vi "Calibration.vi"(0 "Mode":T3, 5 "Calib file":path, 9 "Simulate/Run":T2) -> (14 "Calib const":string[][](array[string]), 16 "Coefficients":dbl[][](array[numeric]) format="%.2f", 19 "Status Out":T1)   [LabVIEW 2013]
uses:
  Anemometry Sub Vis/Globals/Calib_global.vi
  Anemometry Sub Vis/Globals/Meas_global.vi
  Anemometry Sub Vis/Controls/Setup.ctl
  Anemometry Sub Vis/Controls/Post_Process.ctl
  Anemometry Sub Vis/Gen Trav/Multi_Run_Status.ctl
  Anemometry Sub Vis/Controls/App_Global.ctl
  Anemometry Sub Vis/Calibration/Calib_mode.ctl
  Anemometry Sub Vis/Controls/Save_Data.ctl
  Anemometry Sub Vis/Acquisition/PWA/PWAtasksGLOBAL.vi
  Anemometry Sub Vis/File/Setup_Filetype.ctl
  <vilib>/Analysis/NI_AALBase.lvlib
  <vilib>/Analysis/baseanly.llb/Mean (DBL).vi
  Anemometry Sub Vis/Controls/User_Specific_mode.ctl
panel:
  in  "-ve Ref Values":bool
  out "String":string
  in  "polynomial order":i32=2 min=1 max=3 step=1
  out "Ref velocity":dbl[](array[numeric])=[2.4275346736, 2.4395664609, 2.453235235, 2.4247395837, 2.4277603784, 2.41169823, 2.4254144559, 2.424896502176921] format="%.3f"
  out "labels":string[](array[string])=["XW1 Volt", "XW2 Volt", "Entered Val", "Selector"]
  in  "Point selector 3":cluster{"Y":dbl, "X":dbl, "t/f":bool}[](array[cluster]) {"X" format="%#.2g"; "Y" format="%#.3f"}
  in  "n":dbl=0.45 format="%.4f"
  in  "Fixed n":bool=TRUE
  out "Sample of input signals":dbl[][](graph)
  in  "Sampling speeds":T4={"Samples/ch"=600, "Sample Rate/ch (Hz)"=100.0} {"Sample Rate/ch (Hz)" min=0; "Samples/ch" min=0 step=1}
  out "Calibration plot":cluster{cluster{dbl, dbl}[]}[](graph)
  in  "Point selector 4":T5(array[cluster]) {"Y2" format="%#.2f"; "X" format="%#.3f"; "Y" format="%#.2f"}
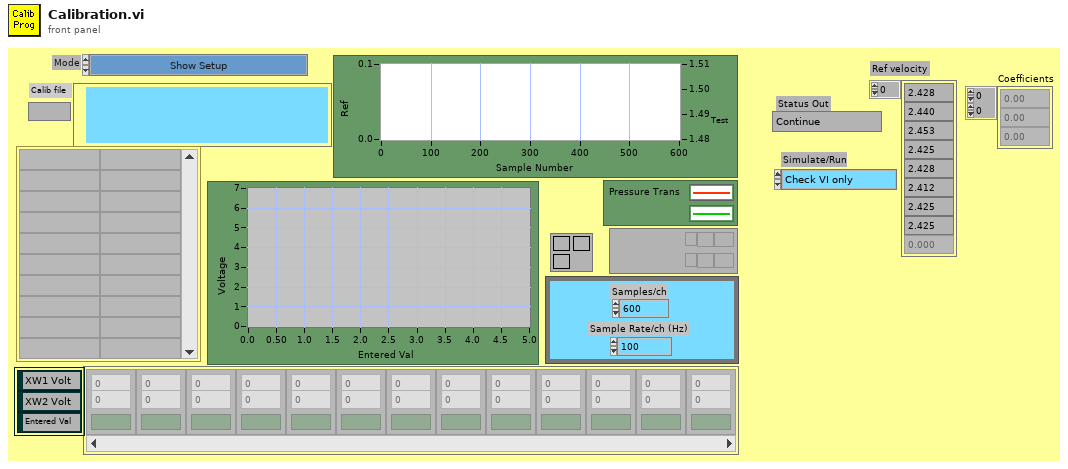
[diagram p1: front panel]
types:
  T1 = typedef "Multi_Run_Status.ctl" = enum16{"Continue", "Jump to Next Point", "Jump to Next Row", "Jump To Fall Back", "Terminate Run"}
  T2 = typedef "User_Specific_mode.ctl" = enum16{"Check VI only", "Run VI"}
  T3 = typedef "Calib_mode.ctl" = enum16{"Show Setup", "Take a New Calibration Point", "Refit Curve", "Setup Front Panel"}
  T4 = cluster{"Samples/ch":i32, "Sample Rate/ch (Hz)":sgl}
  T5 = cluster{"Y":dbl, "Y2":dbl, "X":dbl, "t/f":bool}[]
  T6 = typedef "Post_Process.ctl" = enum16{"Take New Data", "Post Process Raw Data File"}
  T7 = typedef "Setup_Filetype.ctl" = enum16{"Measurement Setups", "Calibration Setups", "General", "Results File Plotter Setups", "Speed Calib Tweaks"}
  T8 = typedef "Save_Data.ctl" = enum16{"Save No Data", "Save Data"}
  T9 = typedef "Setup.ctl" = enum16{"Run Program", "Show Setup", "Save Current Setup", "Setup Front Panel"}
  T10 = typedef "App_Global.ctl" = enum16{"Read Global", "Write to Global", "Initialise Array"}
  T11 = enum32{"existing file", "new file", "new or existing file", "existing dir", "new dir", "new or existing dir", "existing file (use LLBs)", "new file (use LLBs)", "new or existing file (use LLBs)", "new or existing file or directory (use LLBs)"}
  T12 = cluster{"Samples /ch":i32, "Sampling Rate /ch (Hz)":sgl}
  T13 = typedef "Cal_Inst_type.ctl" = enum16{"Propeller anemometer", "Pressure Transducer", "Hot wire", "Cross wire velocity", "Cross wire angle", "Generic Linear", "Generic Polynomial", "Generic BackPoly", "Fast FID", "Thermocouple", "Cold wire", "Pulsed Wire"}
  T14 = typedef "Ref_Inst_type.ctl" = enum16{"Propellor anemometer", "Pressure Transducer", "Raw voltage", "Pitot-static tube", "Preston tube", "Generic Linear", "Generic Polynomial", "Thermocouple", "LDA", "Enter Value", "ADAM Channel"}
  T15 = cluster{"2nd Ref type":T14, "2nd inst present":bool}
  T16 = typedef "Analysis_info_cluster.ctl" = cluster{"Colour":u32, "Inst type":T17, "Inst name":string, "Symbol":string, "Code name":string, "Extra Info":string, "Inst Array":T18, "Extra Titles":string[], "Extra Values":string[], "U":dbl, "u^2":dbl, "u^3":dbl, "u^4":dbl, "Skew_u":dbl, "Kurt_u":dbl, "Sd Error in Mean":dbl, "% u'/U":dbl, "X":dbl, "Y":dbl, "Z":dbl, "Timescale integral to 25%":dbl, "Sd Error in Variance":dbl, "Calib File":path, "Calib Constants":dbl[], "Output Position":bool, "Full Stats":bool, "Av Sampling Rate":dbl, "Av No of Samples":dbl, "Total Meas Time (s)":dbl, "ADAM Ch Name":string}
  T17 = typedef "Inst_type.ctl" = enum16{"Propeller anemometer", "Raw voltage", "Pressure Transducer", "Pitot-static tube", "Preston tube", "Hot wire", "Cross wire 1", "Cross wire 2", "Generic Linear", "Generic Polynomial", "Generic BackPoly", "Fast FID", "Thermocouple", "Cold wire", "Pulsed Wire", "LDA Vel", "LDA Tran time", "LDA Arr time"}
  T18 = typedef "Instrument_Array.ctl" = enum16{"PWA", "LDA", "Analogue"}
  T19 = typedef "Time_Trace_Cluster.ctl" = cluster{"Weighting":dbl[], "Time (s)":dbl[], "Voltage":dbl[], "Eng Values":dbl[]}
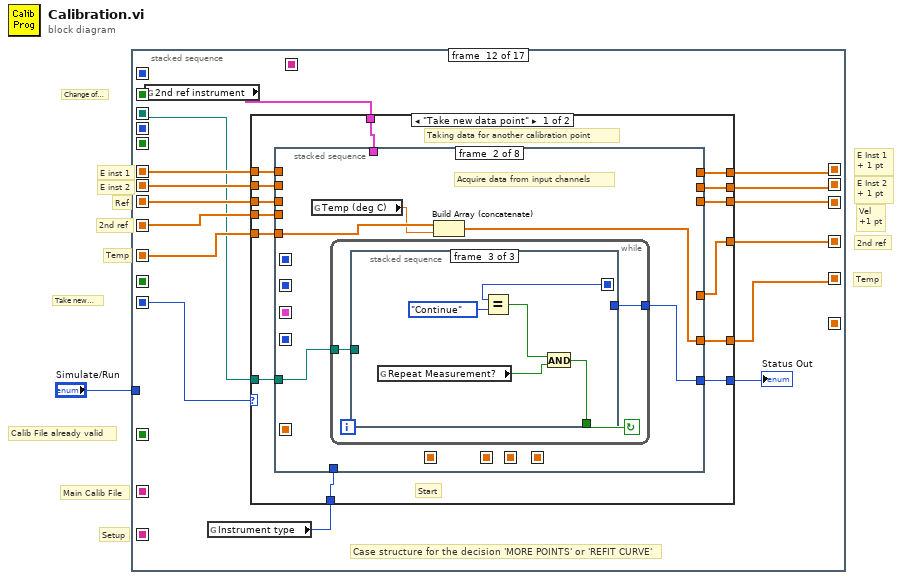
[diagram p0: block diagram]
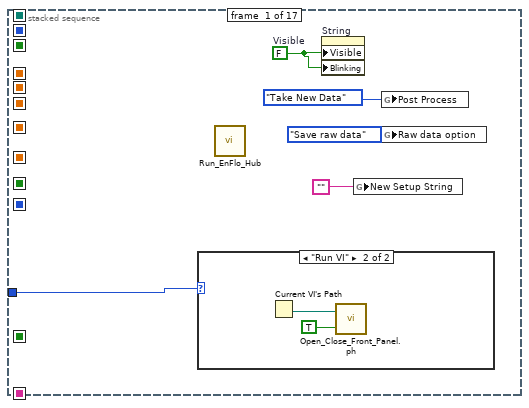
[diagram p2: hidden frame]
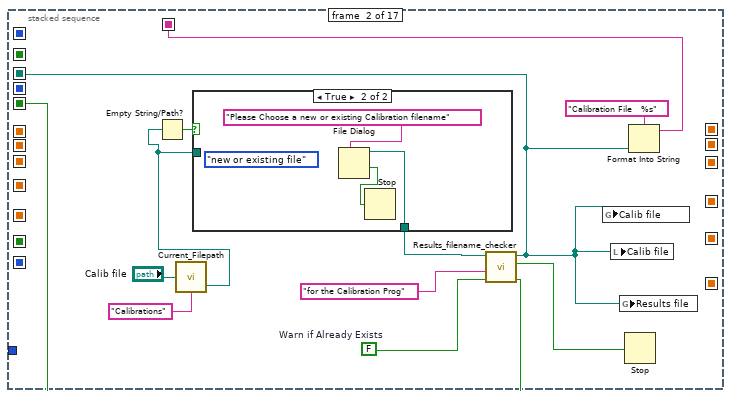
[diagram p4: hidden frame]
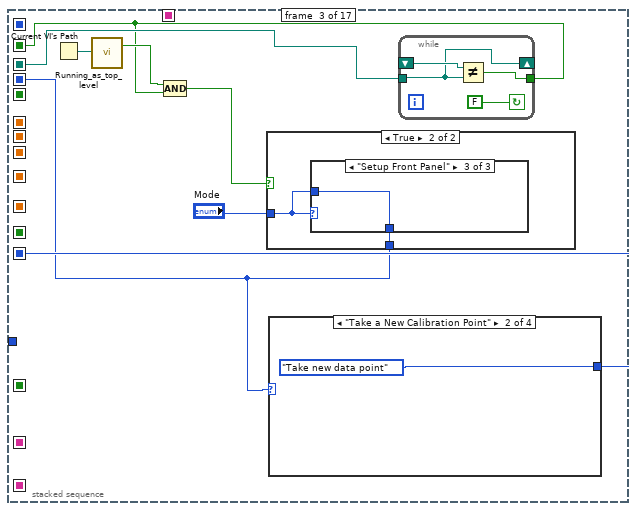
[diagram p6: hidden frame]
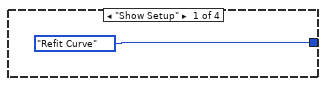
[diagram p7: hidden frame]
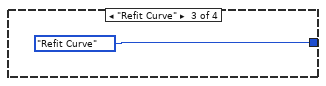
[diagram p8: hidden frame]
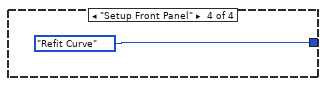
[diagram p9: hidden frame]
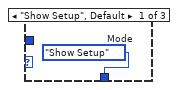
[diagram p11: hidden frame]
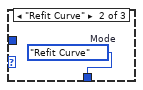
[diagram p12: hidden frame]
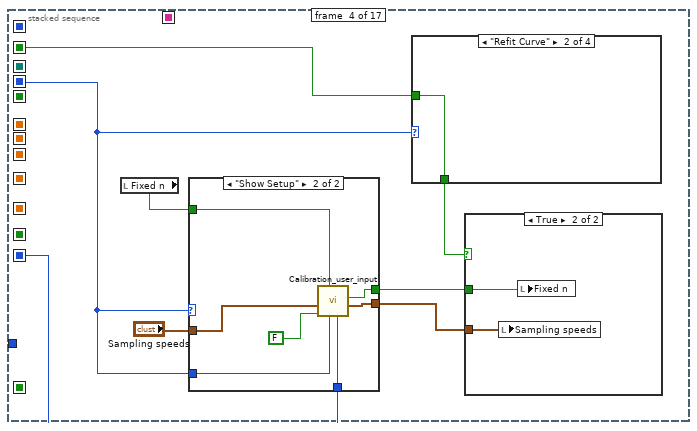
[diagram p13: hidden frame]
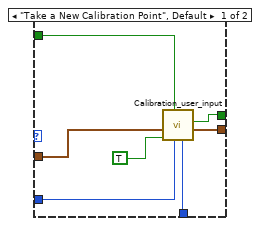
[diagram p14: hidden frame]
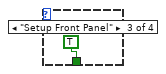
[diagram p16: hidden frame]
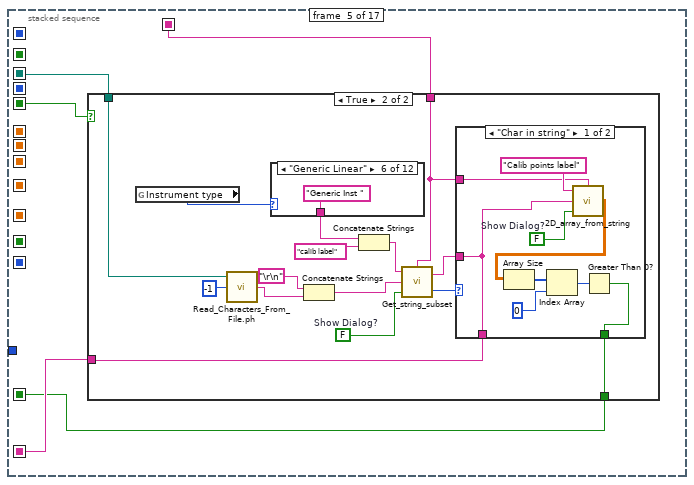
[diagram p19: hidden frame]
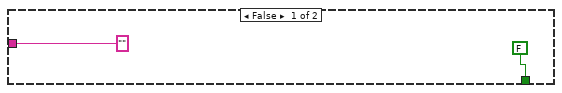
[diagram p20: hidden frame]
diagram:
  # "Change of file"
  # "Take new point"
  # "Calib File already valid"
  # "Main Calib File"
  # "Temp"
  # "Temp"
  # "Setup"
  # "E inst 1"
  # "Ref"
  # "E Inst 1\n+ 1 pt"
  # "Vel\n+1 pt"
  # "E inst 2"
  # "E Inst 2\n+ 1 pt"
  # "2nd ref"
  # "2nd ref"
  n1 = stacked-sequence {
    seq-local: [_ _ _ _ _ _ _ _ _ _ _ w489 _ _ _ _ _] -> [_ _ _ _ _ _ _ _ _ _ _ _ w683 _ _ _ _]
    seq-local: [_ _ _ _ _ _ _ _ _ _ _ w488 _ _ _ _ _] -> [_ _ _ _ _ _ _ _ _ _ _ _ w686 _ _ w749 _]
    seq-local: [_ _ _ _ _ _ _ w376 _ _ _ _ _ _ _ _ _] -> [_ _ _ _ _ _ _ _ _ _ _ w491 _ _ _ _ _]
    seq-local: [_ _ _ _ _ _ _ w375 _ _ _ _ _ _ _ _ _] -> [_ _ _ _ _ _ _ _ _ _ _ w490 _ _ _ _ _]
    seq-local: [_ _ _ _ _ _ _ w374 _ _ _ _ _ _ _ _ _] -> [_ _ _ _ _ _ _ _ _ _ _ w486 _ _ _ _ _]
    seq-local: [_ _ _ _ _ _ _ _ _ _ _ w487 _ _ _ _ _] -> [_ _ _ _ _ _ _ _ _ _ _ _ w685 _ _ _ _]
    seq-local: [_ _ _ _ _ _ _ w373 _ _ _ _ _ _ _ _ _] -> [_ _ _ _ _ _ _ _ _ _ _ w485 _ _ _ _ _]
    seq-local: [_ _ _ _ _ _ _ _ _ _ _ w484 _ _ _ _ _] -> [_ _ _ _ _ _ _ _ _ _ _ _ w680 _ _ _ _]
    seq-local: [_ _ _ _ w78 _ _ _ _ _ _ _ _ _ _ _ _] -> [_ _ _ _ _ _ _ w362 _ _ _ _ _ _ _ _ _]
    seq-local: [_ _ _ _ w79 _ _ _ _ _ _ _ _ _ _ _ _] -> [_ _ _ _ _ _ _ w363 _ _ _ _ _ _ _ _ _]
    seq-local: [_ _ _ _ _ _ _ _ _ _ w464 _ _ _ _ _ _] -> [_ _ _ _ _ _ _ _ _ _ _ _ _ _ w727 _ _]
    seq-local: [_ _ _ _ _ _ _ _ _ _ _ w482 _ _ _ _ _] -> [_ _ _ _ _ _ _ _ _ _ _ _ w684 _ _ _ _]
    seq-local: [_ _ _ _ _ _ _ w372 _ _ _ _ _ _ _ _ _] -> [_ _ _ _ _ _ _ _ _ _ _ w481 _ _ _ _ _]
    seq-local: [_ w13 _ _ _ _ _ _ _ _ _ _ _ _ _ _ _] -> [_ _ w29 _ w77 _ _ _ _ _ w465 w479 _ w709 w736 w750 _]
    seq-local: [_ w18 _ _ _ _ _ _ _ _ _ _ _ _ _ _ _] -> [_ _ _ _ w76 _ _ _ w405 _ _ _ _ _ _ _ _]
    seq-local: [_ _ w32 _ _ _ _ _ _ _ _ _ _ _ _ _ _] -> [_ _ _ w50 _ _ _ _ _ _ _ w478 _ _ _ w751 _]
    seq-local: [_ _ w25 _ _ _ _ _ _ _ _ _ _ _ _ _ _] -> [_ _ _ w49 _ _ _ _ _ w422 _ _ _ _ _ _ w793]
    seq-local: [_ _ _ _ _ _ _ w364 _ _ _ _ _ _ _ _ _] -> [_ _ _ _ _ _ _ _ w403 _ _ _ _ _ _ _ _]
    seq-local: [_ _ _ _ _ _ _ _ _ _ _ _ w681 _ _ _ _] -> [_ _ _ _ _ _ _ _ _ _ _ _ _ w693 _ _ _]
    seq-local: [_ _ _ _ _ _ _ _ _ _ _ _ w679 _ _ _ _] -> [_ _ _ _ _ _ _ _ _ _ _ _ _ w708 _ _ _]
    seq-local: [_ _ w28 _ _ _ _ _ _ _ _ _ _ _ _ _ _] -> [_ _ _ w47 _ _ _ _ w402 _ _ _ _ _ _ _ _]
    seq-local: [_ w12 _ _ _ _ _ _ _ _ _ _ _ _ _ _ _] -> [_ _ _ _ w75 _ _ w357 _ _ _ _ _ _ _ _ _]
    tunnel: "Simulate/Run" -> [w5 _ _ _ _ _ _ _ _ _ _ _ _ _ _ _ _]
    frame #0 {
      w3 = FALSE  # Visible
      n2 = case shown="\"Run VI\"" w5 {
        frame "Check VI only" {
        }
        frame "Run VI" {
          n3 = Current VI's Path() -> (path=w7:path)
          n4 = call "Open_Close_Front_Panel.ph.vi"("Front Panel Window:Open"=TRUE, "VI path"=w7) -> ()  [unwired: 2 out]
        }
      }
      n5 = call "Run_EnFlo_Hub.vi"() -> ()  [unwired: 8 out]
      n6 = property on="String" class="Str"("Visible"=w3, "Blinking"=w3) -> ()  [unwired: 2 in, 2 out]
      n7 = global write "Calib_global.vi" "New Setup String"("") -> ()
      n8 = global write "Meas_global.vi" "Post Process"(Post_Process."Take New Data" ("Post Process")) -> ()
      n9 = global write "Meas_global.vi" "Raw data option"(enum16{"Save raw data", "Raw data not saved"}."Save raw data" ("Raw data option")) -> ()
    }
    frame #1 {
      w19 = FALSE  # Warn if Already Exists
      n10 = call "Current_Filepath.vi"("Filename in"="Calib file", "Data Type"="Calibrations") -> ("Filename Out"=w10:path)  [unwired: 1 out]
      n11 = Empty String/Path?(string/path=w10) -> (empty?=w15:bool)
      n12 = case shown="True" w15 {
        tunnel: w10 -> [w21 _]
        tunnel: [w21 w23] -> w17
        frame False {
        }
        frame True {
          (unwired) T11."new or existing file" ("select mode (2)")
          n13 = File Dialog(7:"Please Choose a new or existing Calibration filename" ("Promp if not found")) -> (1:w22:bool, 3:w23:path)  [unwired: 1 in, 7 out]
          n14 = Stop(stop? (T)=w22) -> ()
        }
      }
      n15 = call "Results_filename_checker.vi"("Warn if Already Exists"=w19, "Comment"="for the Calibration Prog", "Results file"=w17) -> ("exists?"=w18:bool, "cancelled"=w16:bool, "Results file output"=w13:path)  [unwired: 2 in, 1 out]
      n16 = global write "Calib_global.vi" "Calib file"(w13) -> ()
      n17 = local write "Calib file"(w13) -> ()
      n18 = global write "Meas_global.vi" "Results file"(w13) -> ()
      n19 = Stop(stop? (T)=w16) -> ()
      n20 = Format Into String(format string="Calibration File   %s", w13) -> (resulting string=w12:string)  [unwired: 2 in, 1 out]
    }
    frame #2 {
      n21 = Current VI's Path() -> (path=w31:path)
      n22 = call "Running_as_top_level.vi"("Vi path name"=w31) -> ("Top Level"=w30:bool)  [unwired: 1 out]
      n23 = while {
        shift-right: [w45] -> _
        shift-left: _ -> [w46]
        tunnel: w29 -> [w45]
        tunnel: [w44] -> w28
        stop <- FALSE continue-if-true
        n24 = Not Equal?(x=w46, y=w45) -> (x != y?=w44:bool)
      }
      n25 = Compound Arithmetic op=AND(w30, w28) -> (w27:bool)
      n26 = case shown="True" w27 {
        tunnel: "Mode" -> [w37 w38]
        tunnel: [w37 w39] -> w25
        frame False {
        }
        frame True {
          n27 = case shown="\"Setup Front Panel\"" w38 {
            tunnel: [w40 w41 w42] -> w39
            tunnel: w38 -> [_ _ w42]
            frame "Show Setup", Default {
              w40 = Calib_mode."Show Setup"  # Mode
            }
            frame "Refit Curve" {
              w41 = Calib_mode."Refit Curve"  # Mode
            }
            frame "Setup Front Panel" {
            }
          }
        }
      }
      n28 = case shown="\"Take a New Calibration Point\"" w25 {
        tunnel: [enum16{"Take new data point", "Refit Curve"}."Refit Curve" ("data mode") enum16{"Take new data point", "Refit Curve"}."Take new data point" ("data mode") enum16{"Take new data point", "Refit Curve"}."Refit Curve" ("data mode") enum16{"Take new data point", "Refit Curve"}."Refit Curve" ("data mode")] -> w32
        frame "Show Setup" {
        }
        frame "Take a New Calibration Point" {
        }
        frame "Refit Curve" {
        }
        frame "Setup Front Panel" {
        }
      }
    }
    frame #3 {
      n29 = local read "Fixed n"() -> (w52:bool)
      n30 = case shown="\"Show Setup\"" w49 {
        tunnel: "Sampling speeds" -> [w61 w68]
        tunnel: w49 -> [w59 w66]
        tunnel: w50 -> [w58 w65]
        tunnel: [w57 w64] -> w53
        tunnel: w52 -> [w55 w63]
        tunnel: [w56 w62] -> w51
        frame "Take a New Calibration Point", Default {
          n31 = call "Calibration_user_input.vi"("data mode"=w58, "Mode"=w59, "Fixed n"=w55, "OK"=TRUE, "Sampling speeds"=w61) -> ("Sampling speeds Output"=w57:T12, "Fixed n out"=w56:bool)  [unwired: 2 in, 3 out]
        }
        frame "Show Setup" {
          n32 = call "Calibration_user_input.vi"("data mode"=w65, "Mode"=w66, "Fixed n"=w63, "OK"=FALSE, "Sampling speeds"=w68) -> ("Sampling speeds Output"=w64:T12, "Fixed n out"=w62:bool)  [unwired: 5 out]
        }
      }
      n33 = case shown="\"Refit Curve\"" w49 {
        tunnel: [w69 w70 TRUE w72] -> w48
        tunnel: w47 -> [w69 w70 _ w72]
        frame "Show Setup" {
        }
        frame "Refit Curve" {
        }
        frame "Setup Front Panel" {
        }
        frame "Take a New Calibration Point" {
        }
      }
      n34 = case shown="True" w48 {
        tunnel: w53 -> [_ w74]
        tunnel: w51 -> [_ w73]
        frame False {
        }
        frame True {
          n35 = local write "Sampling speeds"(w74) -> ()
          n36 = local write "Fixed n"(w73) -> ()
        }
      }
    }
    frame #4 {
      n37 = case shown="True" w76 {
        tunnel: ["" ("Output string") w96] -> w79
        tunnel: [FALSE w95] -> w78
        tunnel: w77 -> [_ w87]
        tunnel: w75 -> [_ w82]
        frame False {
        }
        frame True {
          w86 = FALSE  # Show Dialog?
          n38 = global read "Calib_global.vi" "Instrument type"() -> (w90:T13)
          n39 = call "Read_Characters_From_File.ph.vi"("file path (dialog if empty)"=w87, "number of characters (all:-1)"=-1) -> ("character string"=w84:string)  [unwired: 7 out]
          n40 = case shown="\"Generic Linear\"" w90 {
            tunnel: ["Prop " "Mano " "HW " "Cross wire velocity " "Cross wire angle " "Generic Inst " "Generic Polynomial " "Generic BackPoly " "Fast FID " "Thermocouple " "Cold wire " "Pulsed wire "] -> w91
            frame "Propeller anemometer" {
            }
            frame "Pressure Transducer" {
            }
            frame "Hot wire" {
            }
            frame "Cross wire velocity" {
            }
            frame "Cross wire angle" {
            }
            frame "Generic Linear" {
            }
            frame "Generic Polynomial" {
            }
            frame "Generic BackPoly" {
            }
            frame "Fast FID" {
            }
            frame "Thermocouple" {
            }
            frame "Cold wire" {
            }
            frame "Pulsed Wire" {
            }
          }
          n41 = Concatenate Strings("\r\n", w84) -> (w83:string)
          n42 = Concatenate Strings(w91, "calib label") -> (w92:string)
          n43 = call "Get_string_subset.vi"("String Name"=w82, "Show Dialog?"=w86, "String to split"=w83, "File Label"=w92) -> ("Status"=w89:enum16{"Char in string", "Char not in string"}, "Output string"=w88:string)
          n44 = case shown="\"Char in string\"" w89 {
            tunnel: w88 -> [w115 _]
            tunnel: [w115 ""] -> w96
            tunnel: [w110 FALSE] -> w95
            tunnel: w82 -> [w109 _]
            frame "Char in string" {
              w116 = FALSE  # Show Dialog?
              n45 = call "2D_array_from_string.vi"("String Name"=w109, "Show Dialog?"=w116, "Input string"=w115, "Array title"="Calib points label") -> ("2D data array"=w114:dbl[][])
              n46 = Array Size(array=w114) -> (size(s)=w113:i32[])
              n47 = Index Array(array=w113, index=0 ("Index")) -> (element=w111:i32)
              n48 = Greater Than 0?(x=w111) -> (x > 0?=w110:bool)
            }
            frame "Char not in string" {
            }
          }
        }
      }
    }
    frame #5 {
      w122 = ""
      n49 = global read "Calib_global.vi" "2nd ref instrument"() -> (w129:T15)
      n50 = global read "Calib_global.vi" "Ref Instrument type"() -> (w130:T14)
      n51 = Unbundle By Name(w129) -> ("2nd Ref type"=w127:T14, "2nd inst present"=w128:bool)
      n52 = global read "Calib_global.vi" "Instrument type"() -> (w133:T13)
      n53 = case shown="\"Propellor anemometer\"" w130 {
        tunnel: [w159 w162 w166 w168 w171 w174 w177 w180 w183 string[] [] string[] []] -> w126
        tunnel: [FALSE FALSE FALSE FALSE TRUE FALSE FALSE FALSE FALSE FALSE FALSE] -> w121
        frame "Propellor anemometer" {
          n54 = Build Array("Prop Velocity") -> (w159:string[])
        }
        frame "Pressure Transducer" {
          n55 = Build Array("Pressure Trans") -> (w162:string[])
        }
        frame "Raw voltage" {
          n56 = Build Array("Raw Voltage") -> (w166:string[])
        }
        frame "Pitot-static tube" {
          n57 = Build Array("Pitot Vel") -> (w168:string[])
        }
        frame "Preston tube" {
          n58 = Build Array("Shear stress") -> (w171:string[])
        }
        frame "Generic Linear" {
          n59 = Build Array("Gen Lin") -> (w174:string[])
        }
        frame "Generic Polynomial" {
          n60 = Build Array("Gen Poly") -> (w177:string[])
        }
        frame "Thermocouple" {
          n61 = Build Array("Thermo") -> (w180:string[])
        }
        frame "LDA" {
          n62 = Build Array("LDA Vel") -> (w183:string[])
        }
        frame "Enter Value" {
        }
        frame "ADAM Channel" {
        }
      }
      n63 = case shown="True" w128 {
        tunnel: w127 -> [_ w136]
        tunnel: [w135 w137] -> w124
        tunnel: w126 -> [w135 _]
        frame False {
        }
        frame True {
          n64 = case shown="\"Propellor anemometer\"" w136 {
            tunnel: [w138 w140 w143 w144 w146 w148 w150 w152 w154 string[] [] string[] []] -> w137
            frame "Propellor anemometer" {
              n65 = Build Array("Prop Velocity") -> (w138:string[])
            }
            frame "Pressure Transducer" {
              n66 = Build Array("Pressure Trans") -> (w140:string[])
            }
            frame "Raw voltage" {
              n67 = Build Array("Raw Voltage") -> (w143:string[])
            }
            frame "Pitot-static tube" {
              n68 = Build Array("Pitot Vel") -> (w144:string[])
            }
            frame "Preston tube" {
              n69 = Build Array("Shear stress") -> (w146:string[])
            }
            frame "Generic Linear" {
              n70 = Build Array("Gen Lin") -> (w148:string[])
            }
            frame "Generic Polynomial" {
              n71 = Build Array("Gen Poly") -> (w150:string[])
            }
            frame "Thermocouple" {
              n72 = Build Array("Thermo") -> (w152:string[])
            }
            frame "LDA" {
              n73 = Build Array("LDA Vel") -> (w154:string[])
            }
            frame "Enter Value" {
            }
            frame "ADAM Channel" {
            }
          }
        }
      }
      n74 = case shown="\"Pulsed Wire\"" w133 {
        tunnel: [w193 w197 w201 w205 w210 w215 w219 w223 w227 w231 w235 w240] -> w123
        tunnel: [FALSE FALSE FALSE FALSE FALSE FALSE TRUE TRUE FALSE FALSE TRUE TRUE] -> w125
        tunnel: [w191 w195 w199 w203 w208 w213 w217 w221 w225 w229 w233 FALSE] -> w120
        tunnel: w121 -> [w191 w195 w199 w203 w208 w213 w217 w221 w225 w229 w233 _]
        frame "Propeller anemometer" {
          n75 = Build Array("Prop Voltage") -> (w193:string[])
        }
        frame "Pressure Transducer" {
          n76 = Build Array("Pressure Trans") -> (w197:string[])
        }
        frame "Hot wire" {
          n77 = Build Array("HW Voltage") -> (w201:string[])
        }
        frame "Cross wire velocity" {
          n78 = Build Array("XW1 Voltage", "XW2 Voltage") -> (w205:string[])
        }
        frame "Cross wire angle" {
          n79 = Build Array("XW1 Voltage", "XW2 Voltage") -> (w210:string[])
        }
        frame "Generic Linear" {
          n80 = Build Array("Generic Voltage") -> (w215:string[])
        }
        frame "Generic Polynomial" {
          n81 = Build Array("Generic Voltage") -> (w219:string[])
        }
        frame "Generic BackPoly" {
          n82 = Build Array("Generic Voltage") -> (w223:string[])
        }
        frame "Fast FID" {
          n83 = Build Array("FF Voltage") -> (w227:string[])
        }
        frame "Thermocouple" {
          n84 = Build Array("Thermo Voltage") -> (w231:string[])
        }
        frame "Cold wire" {
          n85 = Build Array("CW Voltage") -> (w235:string[])
        }
        frame "Pulsed Wire" {
          n86 = local write "polynomial order"(3 ("polynomial order")) -> ()
          n87 = Build Array("PWA 1/TOF") -> (w240:string[])
        }
      }
      n88 = property on="polynomial order" class="DigNum (strict)"("Visible"=w125) -> ()  [unwired: 2 in, 2 out]
      n89 = Build Array (concatenate)(w124, w123, w122, w122, w122) -> (w131:string[])
      n90 = for {
        N: 3 -> [_]
        tunnel: w131 -> [w189] mode=indexing
        i -> [w190]
        n91 = property on="Sample of input signals" class="WFGraph (strict)"("Active Plot"=w190, "Plot.Plot Name"=w189) -> ()  [unwired: 2 in, 2 out]
      }
      n92 = case shown="False" w120 {
        frame False {
          n93 = local write "-ve Ref Values"(FALSE ("-ve Ref Values")) -> ()
        }
        frame True {
        }
      }
      n94 = property on="-ve Ref Values" class="Bool (strict)"("Visible"=w120) -> ()  [unwired: 2 in, 2 out]
    }
    frame #6 {
      n95 = global read "Calib_global.vi" "Instrument type"() -> (w245:T13)
      n96 = global read "Calib_global.vi" "Ref Instrument type"() -> (w244:T14)
      n97 = case shown="\"Propellor anemometer\"" w244 {
        tunnel: ["Prop Vel" "Pressure" "Voltage" "Pitot Vel" "Shear stress" "Generic Linear" "Generic Poly" "Thermo T" "LDA Vel" "Entered Val" "ADAM Channel"] -> w247
        frame "Propellor anemometer" {
        }
        frame "Pressure Transducer" {
        }
        frame "Raw voltage" {
        }
        frame "Pitot-static tube" {
        }
        frame "Preston tube" {
        }
        frame "Generic Linear" {
        }
        frame "Generic Polynomial" {
        }
        frame "Thermocouple" {
        }
        frame "LDA" {
        }
        frame "Enter Value" {
        }
        frame "ADAM Channel" {
        }
      }
      n98 = case shown="\"Cross wire velocity\"" w245 {
        tunnel: [FALSE FALSE TRUE TRUE TRUE FALSE FALSE FALSE FALSE FALSE FALSE FALSE] -> w250
        tunnel: [TRUE TRUE TRUE FALSE FALSE TRUE TRUE TRUE TRUE TRUE TRUE TRUE] -> w249
        tunnel: [FALSE FALSE FALSE TRUE TRUE FALSE FALSE FALSE FALSE FALSE FALSE FALSE] -> w248
        tunnel: w247 -> [w252 w259 w268 w278 w288 w298 w304 w311 w318 w326 w332 w339]
        tunnel: [w255 w262 w271 w281 w291 w300 w307 w314 w321 w328 w335 w342] -> w246
        tunnel: "Selector" -> [w254 w261 w270 w280 w290 w297 w306 w313 w320 w325 w334 w341]
        tunnel: [w253 w260 "E^2" "XW Volt^2" "Y" w299 w304 w312 w318 w327 w332 w339] -> w242
        tunnel: [w252 w259 w266 w276 "X" w298 w305 w311 w319 w326 w333 w340] -> w243
        frame "Propeller anemometer" {
          w253 = "Prop Volt"
          n99 = Build Array(w253, w252, w254) -> (w255:string[])
        }
        frame "Pressure Transducer" {
          w260 = "Voltage"
          n100 = Build Array(w260, w259, w261) -> (w262:string[])
        }
        frame "Hot wire" {
          n101 = Build Array("HW Volt", w268, w270) -> (w271:string[])
          n102 = Concatenate Strings(w268, "^n") -> (w266:string)
        }
        frame "Cross wire velocity" {
          n103 = Build Array("XW1 Volt", "XW2 Volt", w278, w280) -> (w281:string[])
          n104 = Concatenate Strings(w278, "^n") -> (w276:string)
        }
        frame "Cross wire angle" {
          n105 = Build Array("XW1 Volt", "XW2 Volt", w288, w290) -> (w291:string[])
        }
        frame "Generic Linear" {
          w299 = "Gen Volt"
          n106 = Build Array(w299, w298, w297) -> (w300:string[])
        }
        frame "Generic Polynomial" {
          w305 = "Gen Volt"
          n107 = Build Array(w305, w304, w306) -> (w307:string[])
        }
        frame "Generic BackPoly" {
          w312 = "Gen Volt"
          n108 = Build Array(w311, w312, w313) -> (w314:string[])
        }
        frame "Fast FID" {
          w319 = "FF Volt"
          n109 = Build Array(w319, w318, w320) -> (w321:string[])
        }
        frame "Thermocouple" {
          w327 = "Thermo Volt"
          n110 = Build Array(w327, w326, w325) -> (w328:string[])
        }
        frame "Cold wire" {
          w333 = "CW Volt"
          n111 = Build Array(w333, w332, w334) -> (w335:string[])
        }
        frame "Pulsed Wire" {
          w340 = "1/TOF"
          n112 = Build Array(w340, w339, w341) -> (w342:string[])
        }
      }
      "labels" <- w246
      n113 = property on="n" class="DigNum (strict)"("Visible"=w250) -> ()  [unwired: 2 in, 2 out]
      n114 = property on="Fixed n" class="Bool (strict)"("Visible"=w250) -> ()  [unwired: 2 in, 2 out]
      n115 = property on="Calibration plot" class="XYGraph (strict)"("X Scale.Name Label.Text"=w243, "Y Scale.Name Label.Text"=w242) -> ()  [unwired: 2 in, 2 out]
      n116 = property on="Point selector 3" class="Arr (strict)"("Visible"=w249) -> ()  [unwired: 2 in, 2 out]
      n117 = property on="Point selector 4" class="Arr (strict)"("Visible"=w248) -> ()  [unwired: 2 in, 2 out]
    }
    frame #7 {
      # "Case structure to read previous calibration points if required"
      n118 = global read "Calib_global.vi" "Calibration Points"() -> (w361:dbl[])
      n119 = case shown="True" w362 {
        tunnel: w363 -> [_ w396]
        tunnel: [w388 w393] -> w360
        tunnel: w361 -> [w389 w392]
        tunnel: w357 -> [_ w390]
        frame False {
          n120 = Build Array(w389) -> (w388:dbl[][])
        }
        frame True {
          w395 = FALSE  # Show Dialog?
          n121 = Array Size(array=w392) -> (size(s)=w391:i32)
          n122 = call "2D_array_from_string.vi"("String Name"=w390, "Show Dialog?"=w395, "Input string"=w396, "Array title"="Calib points label") -> ("2D data array"=w394:dbl[][])
          n123 = case shown="0" w391 {
            tunnel: w394 -> [w398 w401]
            tunnel: [w398 w400] -> w393
            tunnel: w392 -> [_ w399]
            frame 0 {
            }
            frame 1, Default {
              n124 = Build Array (concatenate)(w401, w399) -> (w400:dbl[][])
            }
          }
        }
      }
      n125 = for {
        tunnel: w360 -> [w378] mode=indexing
        shift-right: [w377] -> w358
        shift-left: dbl[][] [] -> [w379]
        n126 = Array Subset(array=w378, length=2) -> (w382:dbl[])  [unwired: 1 in]
        n127 = Not A Number/Path/Refnum?(number/path/refnum=w382) -> (NaN/Path/Refnum?=w381:bool[])
        n128 = Or Array Elements(Boolean array=w381) -> (logical OR=w380:bool)
        n129 = case shown="False" w380 {
          tunnel: w379 -> [w386 w387]
          tunnel: w378 -> [w385 _]
          tunnel: [w384 w387] -> w377
          frame False {
            n130 = Build Array (concatenate)(w386, w385) -> (w384:dbl[][])
          }
          frame True {
          }
        }
      }
      n131 = Index Array(array=w358, index (col)=0) -> (element=w375:dbl[])  [unwired: 1 in]
      n132 = Index Array(array=w358, index (col)=1) -> (element=w376:dbl[])  [unwired: 1 in]
      n133 = Index Array(array=w358, index (col)=2) -> (element=w374:dbl[])  [unwired: 1 in]
      n134 = Index Array(array=w358, index (col)=3) -> (element=w373:dbl[])  [unwired: 1 in]
      n135 = Index Array(array=w358, index (col)=4) -> (element=w372:dbl[])  [unwired: 1 in]
      n136 = Index Array(array=w358, index (col)=5) -> (element=w365:dbl[])  [unwired: 1 in]
      n137 = Not A Number/Path/Refnum?(number/path/refnum=w365) -> (NaN/Path/Refnum?=w364:bool[])
    }
    frame #8 {
      n138 = And(x=w402, y=w405) -> (x .and. y?=w404:bool)
      n139 = case shown="True" w404 {
        tunnel: w403 -> [_ w406]
        frame False {
        }
        frame True {
          n140 = local read "Point selector 3"() -> (w410:cluster{"Y":dbl, "X":dbl, "t/f":bool}[])
          n141 = local read "Point selector 4"() -> (w407:T5)
          n142 = for {
            tunnel: w410 -> [w418]
            tunnel: [w420] -> w409 mode=indexing
            tunnel: w406 -> [w419] mode=indexing
            i -> [w417]
            n143 = Index Array(array=w418, index=w417) -> (element=w416:cluster{"Y":dbl, "X":dbl, "t/f":bool})
            n144 = Bundle By Name(cluster=w416, "t/f"=w419) -> (w420:cluster{"Y":dbl, "X":dbl, "t/f":bool})
          }
          n145 = for {
            tunnel: w407 -> [w413]
            tunnel: [w415] -> w408 mode=indexing
            tunnel: w406 -> [w414] mode=indexing
            i -> [w412]
            n146 = Index Array(array=w413, index=w412) -> (element=w411:cluster{"Y":dbl, "Y2":dbl, "X":dbl, "t/f":bool})
            n147 = Bundle By Name(cluster=w411, "t/f"=w414) -> (w415:cluster{"Y":dbl, "Y2":dbl, "X":dbl, "t/f":bool})
          }
          n148 = local write "Point selector 3"(w409) -> ()
          n149 = local write "Point selector 4"(w408) -> ()
        }
      }
    }
    frame #9 {
      w425 = "Setup for instrument being calibrated"
      n150 = global read "Calib_global.vi" "Pre Setup String"() -> (w423:string)
      n151 = case shown="\"Show Setup\"" w422 {
        tunnel: w423 -> [w430 w434]
        tunnel: w425 -> [w429 w433]
        tunnel: [w428 w432] -> w424
        tunnel: "Previous Setup String" ("String Name") -> [w427 w431]
        frame "Take a New Calibration Point", Default {
          n152 = call "Get_string_subset.vi"("String Name"=w427, "String to split"=w430, "File Label"=w429) -> ("Output string"=w428:string)  [unwired: 1 in, 1 out]
        }
        frame "Show Setup" {
          n153 = global read "Calib_global.vi" "Instrument type"() -> (w438:T13)
          n154 = call "Get_string_subset.vi"("String Name"=w431, "String to split"=w434, "File Label"=w433) -> ("Status"=w436:enum16{"Char in string", "Char not in string"}, "Output string"=w437:string)  [unwired: 1 in]
          n155 = case shown="\"Char in string\"" w436 {
            tunnel: [w459 w460] -> w435
            tunnel: w437 -> [w459 _]
            tunnel: w434 -> [_ w460]
            frame "Char in string" {
            }
            frame "Char not in string" {
            }
          }
          n156 = case shown="\"Propeller anemometer\"" w438 {
            tunnel: [w440 w442 w445 w448 w451 w453 w455 w457 ""] -> w432
            tunnel: w435 -> [w439 w441 w443 w446 w449 w452 w454 w456 _]
            frame "Propeller anemometer" {
              n157 = call "Propeller_setup.vi"("Setup String"=w439) -> ("Output string"=w440:string)
            }
            frame "Pressure Transducer" {
              n158 = call "Pressure_Transducer_Setup.vi"("Setup String"=w441) -> ("Output string"=w442:string)
            }
            frame "Hot wire" {
              n159 = call "Hot_Wire_Setup.vi"("XW?"=FALSE, "Setup String"=w443) -> ("Output string"=w445:string)
            }
            frame "Cross wire velocity" {
              n160 = call "Hot_Wire_Setup.vi"("XW?"=TRUE, "Setup String"=w446) -> ("Output string"=w448:string)
            }
            frame "Cross wire angle" {
              n161 = call "Hot_Wire_Setup.vi"("XW?"=TRUE, "Setup String"=w449) -> ("Output string"=w451:string)
            }
            frame "Generic Linear" {
              n162 = call "Generic_setup.vi"("Setup String"=w452) -> ("Output String"=w453:string)
            }
            frame "Generic Polynomial" {
              n163 = call "Generic_setup.vi"("Setup String"=w454) -> ("Output String"=w455:string)
            }
            frame "Generic BackPoly" {
              n164 = call "Generic_setup.vi"("Setup String"=w456) -> ("Output String"=w457:string)
            }
            frame "Fast FID", Default {
            }
          }
        }
      }
      n165 = call "Add_label_to_string.vi"("String to write"=w424, "File Label"=w425) -> ("Output string"=w426:string)
      n166 = global write "Calib_global.vi" "Instument setup Info"(w426) -> ()
    }
    frame #10 {
      w466 = TRUE  # Lock File
      w472 = FALSE  # advisory dialog? (display:T)
      w473 = FALSE  # append to file? (new file:F)
      n167 = Path To String(path=w465) -> (string=w467:string)
      n168 = global read "Calib_global.vi" "Instument setup Info"() -> (w468:string)
      n169 = global read "Calib_global.vi" "New Setup String"() -> (w469:string)
      n170 = call "Date_and_Time_to_string.vi"() -> ("Date and time (spreadsheet)"=w475:string)
      n171 = call "Characters_to_string.vi"("Characters to write"=w467, "Label for characters"="Calib filename") -> ("Output string"=w476:string)
      n172 = Concatenate Strings(w475, w476, w469, w468) -> (w464:string)
      n173 = call "Add_label_to_string.vi"("String to write"=w464, "File Label"="Raw data header") -> ("Output string"=w470:string)
      n174 = call "Setup_Filepath.vi"("Setup File Type"=Setup_Filetype."Calibration Setups", "Filename in"="Current_Setup.xls") -> ("Filename Out"=w461:path)  [unwired: 1 out]
      n175 = call "Calib_read_files.vi"() -> ()  [unwired: 1 out]
      n176 = call "Write_Characters_To_File.vi"("file path (dialog if empty)"=w461, "advisory dialog? (display:T)"=w472, "character string"=w470, "append to file? (new file:F)"=w473, "Lock File"=w466) -> ()  [unwired: 4 out]
    }
    frame #11 {
      # "Case structure for the decision 'MORE POINTS' or 'REFIT CURVE'"
      n177 = global read "Calib_global.vi" "2nd ref instrument"() -> (w483:T15)
      n178 = global read "Calib_global.vi" "Instrument type"() -> (w477:T13)
      n179 = case shown="\"Take new data point\"" w478 {
        tunnel: [w502 w678] -> w488
        tunnel: [w503 w674] -> w489
        tunnel: w491 -> [w504 w678]
        tunnel: w490 -> [w505 w674]
        tunnel: [w501 w677] -> w487
        tunnel: w486 -> [w500 w677]
        tunnel: w485 -> [w499 w676]
        tunnel: [w497 w676] -> w484
        tunnel: w483 -> [w498 _]
        tunnel: [w495 w675] -> w482
        tunnel: w481 -> [w496 w675]
        tunnel: w479 -> [w494 _]
        tunnel: [w493 Multi_Run_Status."Continue" ("Status Out")] -> w480
        tunnel: w477 -> [w492 _]
        frame "Take new data point" {
          # "Start"
          # "Taking data for another calibration point"
          n180 = stacked-sequence {
            seq-local: [_ _ _ _ w569 _ _ _] -> [_ _ _ _ _ w587 _ _]
            seq-local: [w509 _ _ _ _ _ _ _] -> [_ _ _ _ w570 w580 _ _]
            seq-local: [_ _ w535 _ _ _ _ _] -> [_ _ _ _ _ _ w611 _]
            seq-local: [_ _ _ _ _ w579 _ _] -> [_ _ _ _ _ _ w610 _]
            seq-local: [_ _ w533 _ _ _ _ _] -> [_ _ _ _ _ w578 w609 _]
            seq-local: [_ _ _ w550 _ _ _ _] -> [_ _ _ _ w565 _ _ _]
            seq-local: [_ _ _ w548 _ _ _ _] -> [_ _ _ _ _ _ w607 _]
            seq-local: [_ _ _ w547 _ _ _ _] -> [_ _ _ _ _ _ w606 _]
            seq-local: [_ _ _ w546 _ _ _ _] -> [_ _ _ _ _ w576 _ _]
            tunnel: w504 -> [_ _ _ _ _ _ w615 _]
            tunnel: [_ _ _ _ w572 _ _ _] -> w503
            tunnel: w505 -> [_ _ _ _ w571 _ _ _]
            tunnel: [_ _ _ _ _ _ w614 _] -> w502
            tunnel: [_ _ _ _ _ _ w613 _] -> w501
            tunnel: w500 -> [_ _ _ _ _ _ w612 _]
            tunnel: w499 -> [_ _ _ _ _ w583 _ _]
            tunnel: [_ _ _ _ _ w582 _ _] -> w497
            tunnel: w498 -> [_ _ _ _ _ w581 _ _]
            tunnel: w496 -> [_ w514 _ _ _ _ _ _]
            tunnel: [_ w513 _ _ _ _ _ _] -> w495
            tunnel: w494 -> [_ w511 _ _ _ _ _ _]
            tunnel: [_ w512 _ _ _ _ _ _] -> w493
            tunnel: w492 -> [_ _ _ w549 _ w577 w608 _]
            frame #0 {
              w506 = TRUE  # Visible
              w507 = "Current Taking a New Calibration Point"  # String
              n181 = Get Date/Time In Seconds() -> (seconds since 1Jan1904=w508:timestamp)
              n182 = To Double Precision Float(number=w508) -> (double precision float=w509:dbl)
              n183 = property on="String" class="Str"("Visible"=w506, "Blinking"=w506) -> ()  [unwired: 2 in, 2 out]
              "String" <- w507
            }
            frame #1 {
              # "Acquire data from input channels"
              n184 = global read "Calib_global.vi" "Temp (deg C)"() -> (w510:dbl)
              n185 = while {
                tunnel: [w517] -> w512
                tunnel: w511 -> [w516]
                stop <- w515 continue-if-true
                n186 = stacked-sequence {
                  seq-local: [_ w519 _] -> [_ _ w527]
                  tunnel: [_ w519 _] -> w517
                  tunnel: w516 -> [_ w523 _]
                  tunnel: [_ _ w528] -> w515
                  frame #0 {
                    n187 = global write "Meas_global.vi" "Remote control"(TRUE ("Remote control")) -> ()
                  }
                  frame #1 {
                    n188 = call "Get_Data_Base_file_code.vi"("Results Filename"=w523, "Data Type"="Raw_Calibrations") -> ("Raw Data File Name"=w520:path)  [unwired: 3 out]
                    n189 = call "Measurement.vi"("setup"=Setup."Run Program", "Post Process"=Post_Process."Take New Data", "File"=Save_Data."Save No Data", "Raw data file"=w520, "Setup filename"="Calib_Setup.xls") -> ("Status Out"=w519:T1)  [unwired: 2 in, 12 out]
                  }
                  frame #2 {
                    n190 = global read "Meas_global.vi" "Repeat Measurement?"() -> (w529:bool)
                    n191 = Equal?(x=w527, y=Multi_Run_Status."Continue" ("Status Out")) -> (x = y?=w530:bool)
                    n192 = And(x=w530, y=w529) -> (x .and. y?=w528:bool)
                  }
                }
              }
              n193 = Build Array (concatenate)(w514, w510) -> (w513:dbl[])
            }
            frame #2 {
              n194 = global read "Meas_global.vi" "Analysis Info cluster"() -> (w535:T16[])
              n195 = global read "Meas_global.vi" "Time Trace"() -> (w532:T19[])
              n196 = for {
                tunnel: w535 -> [w541] mode=indexing
                shift-right: [w538] -> w533
                shift-left: dbl[][] [] -> [w539]
                tunnel: w532 -> [w537] mode=indexing
                n197 = Unbundle By Name(w537) -> ("Eng Values"=w536:dbl[])
                n198 = Unbundle By Name(w541) -> ("Inst Array"=w540:T18)
                n199 = case shown="\"PWA\", Default" w540 {
                  tunnel: w539 -> [w542 w545]
                  tunnel: w536 -> [_ w544]
                  tunnel: [w542 w543] -> w538
                  frame "PWA", Default {
                  }
                  frame "Analogue" {
                    n200 = Build Array (concatenate)(w545, w544) -> (w543:dbl[][])
                  }
                }
              }
              "Sample of input signals" <- w533
            }
            frame #3 {
              n201 = case shown="\"Pulsed Wire\"" w549 {
                tunnel: [0 ("Index in") 1 ("Index in")] -> w550
                tunnel: [w551 w554] -> w548
                tunnel: [w551 w558] -> w547
                tunnel: [w551 w557] -> w546
                frame "Propeller anemometer", Default {
                  w551 = 0.0 ("mean")
                }
                frame "Pulsed Wire" {
                  n202 = global read "PWAtasksGLOBAL.vi" "PWA 1/TOF"() -> (w561:dbl[][])
                  n203 = Index Array(array=w561, index (row)=0) -> (element=w559:dbl[])  [unwired: 1 in]
                  n204 = call "Mean_fr_NaN_data.vi"("Data"=w559) -> ("Mean value"=w554:dbl)  [unwired: 1 out]
                  n205 = Less Than 0?(x=w554) -> (x < 0?=w553:bool)
                  n206 = local write "-ve Ref Values"(w553) -> ()
                  n207 = Multiply(x=w559, y=w559) -> (x*y=w556:dbl[])
                  n208 = call "Mean_fr_NaN_data.vi"("Data"=w556) -> ("Mean value"=w558:dbl)  [unwired: 1 out]
                  n209 = Multiply(x=w559, y=w556) -> (x*y=w555:dbl[])
                  n210 = call "Mean_fr_NaN_data.vi"("Data"=w555) -> ("Mean value"=w557:dbl)  [unwired: 1 out]
                }
              }
            }
            frame #4 {
              # "Adding the velocity value to the array"
              n211 = global read "Calib_global.vi" "ADAM Channel Name"() -> (w563:string)
              n212 = global read "Calib_global.vi" "Ref Instrument type"() -> (w568:T14)
              n213 = call "Get_ref_inst_value.vi"("Ref Instrument type"=w568, "ADAM Channel Name"=w563, "Index in"=w565, "Start time"=w570) -> ("Ref Value"=w567:dbl, "Index out"=w569:i32)  [unwired: 3 in, 7 out]
              n214 = case shown="True" "-ve Ref Values" {
                tunnel: w567 -> [w573 w575]
                tunnel: [w573 w574] -> w566
                frame False {
                }
                frame True {
                  n215 = Negate(x=w575) -> (-x=w574:dbl)
                }
              }
              n216 = Build Array (concatenate)(w571, w566) -> (w572:dbl[])
            }
            frame #5 {
              n217 = Unbundle(w581) -> ("2nd Ref type"=w585:T14, "2nd inst present"=w584:bool)
              n218 = case shown="True" w584 {
                tunnel: w587 -> [w592 w602]
                tunnel: [w590 w603] -> w586
                tunnel: w585 -> [_ w604]
                tunnel: w580 -> [_ w605]
                tunnel: [w592 w601] -> w579
                tunnel: w578 -> [w591 _]
                tunnel: w577 -> [w589 _]
                tunnel: w576 -> [w588 _]
                frame False {
                  n219 = case shown="\"Generic Polynomial\"" w589 {
                    tunnel: w592 -> [_ w598 _]
                    tunnel: w591 -> [_ w597 _]
                    tunnel: [0.0 ("mean") w595 w599] -> w590
                    tunnel: w588 -> [_ _ w599]
                    frame "Propeller anemometer", Default {
                    }
                    frame "Generic Polynomial" {
                      n220 = Index Array(array=w597, index (row)=w598) -> (element=w594:dbl[])  [unwired: 1 in]
                      n221 = Compound Arithmetic op=MULTIPLY(w594, w594, w594) -> (w596:dbl[])
                      n222 = call-poly <vilib>:"Mean.vi"("X"=w596) -> ("mean"=w595:dbl)  [unwired: 1 out]
                    }
                    frame "Pulsed Wire" {
                    }
                  }
                }
                frame True {
                  n223 = global read "Calib_global.vi" "ADAM Channel Name Vel Ref"() -> (w600:string)
                  n224 = call "Get_ref_inst_value.vi"("Ref Instrument type"=w604, "ADAM Channel Name"=w600, "Index in"=w602, "Start time"=w605) -> ("Ref Value"=w603:dbl, "Index out"=w601:i32)  [unwired: 4 in, 6 out]
                }
              }
              n225 = Build Array (concatenate)(w583, w586) -> (w582:dbl[])
            }
            frame #6 {
              n226 = case shown="\"Generic Polynomial\"" w608 {
                tunnel: w615 -> [w620 w630 w637 w645 w657 w668]
                tunnel: [w621 w631 w638 w646 w658 w669] -> w614
                tunnel: w612 -> [w619 w629 w636 w641 w656 w667]
                tunnel: [w619 w628 w635 w639 w655 w666] -> w613
                tunnel: w611 -> [w617 _ _ w643 w651 w662]
                tunnel: w610 -> [w622 w632 _ w647 w649 w660]
                tunnel: w609 -> [_ w627 _ _ _ _]
                tunnel: w607 -> [_ _ w634 _ _ _]
                tunnel: w606 -> [_ _ w633 _ _ _]
                frame "Propeller anemometer", Default {
                  n227 = Index Array(array=w617, index=w622) -> (element=w618:T16)
                  n228 = Unbundle By Name(w618) -> ("U"=w616:dbl)
                  n229 = Build Array (concatenate)(w620, w616) -> (w621:dbl[])
                }
                frame "Generic Polynomial" {
                  n230 = Index Array(array=w627, index (row)=w632) -> (element=w624:dbl[])  [unwired: 1 in]
                  n231 = call-poly <vilib>:"Mean.vi"("X"=w624) -> ("mean"=w626:dbl)  [unwired: 1 out]
                  n232 = Multiply(x=w624, y=w624) -> (x*y=w623:dbl[])
                  n233 = call-poly <vilib>:"Mean.vi"("X"=w623) -> ("mean"=w625:dbl)  [unwired: 1 out]
                  n234 = Build Array (concatenate)(w630, w626) -> (w631:dbl[])
                  n235 = Build Array (concatenate)(w629, w625) -> (w628:dbl[])
                }
                frame "Pulsed Wire" {
                  n236 = Build Array (concatenate)(w637, w634) -> (w638:dbl[])
                  n237 = Build Array (concatenate)(w636, w633) -> (w635:dbl[])
                }
                frame "Fast FID" {
                  n238 = Index Array(array=w643, index=w647) -> (element=w644:T16)
                  n239 = Unbundle By Name(w644) -> ("U"=w642:dbl, "u^2"=w640:dbl)
                  n240 = Build Array (concatenate)(w645, w642) -> (w646:dbl[])
                  n241 = Build Array (concatenate)(w641, w640) -> (w639:dbl[])
                }
                frame "Cross wire velocity" {
                  n242 = Increment(x=w649) -> (x+1=w648:i32)
                  n243 = Index Array(array=w651, index=w649) -> (element=w654:T16)
                  n244 = Index Array(array=w651, index=w648) -> (element=w653:T16)
                  n245 = Unbundle By Name(w654) -> ("U"=w650:dbl)
                  n246 = Unbundle By Name(w653) -> ("U"=w652:dbl)
                  n247 = Build Array (concatenate)(w657, w650) -> (w658:dbl[])
                  n248 = Build Array (concatenate)(w656, w652) -> (w655:dbl[])
                }
                frame "Cross wire angle" {
                  n249 = Increment(x=w660) -> (x+1=w659:i32)
                  n250 = Index Array(array=w662, index=w660) -> (element=w665:T16)
                  n251 = Index Array(array=w662, index=w659) -> (element=w664:T16)
                  n252 = Unbundle By Name(w665) -> ("U"=w661:dbl)
                  n253 = Unbundle By Name(w664) -> ("U"=w663:dbl)
                  n254 = Build Array (concatenate)(w668, w661) -> (w669:dbl[])
                  n255 = Build Array (concatenate)(w667, w663) -> (w666:dbl[])
                }
              }
            }
            frame #7 {
              w670 = FALSE  # Visible
              n256 = global read "Meas_global.vi" "Raw data file"() -> (w672:path)
              n257 = Strip Path(path=w672) -> (stripped path=w671:path)  [unwired: 1 out]
              n258 = global write "Calib_global.vi" "Calib Raw Data Folder"(w671) -> ()
              n259 = property on="String" class="Str"("Visible"=w670, "Blinking"=w670) -> ()  [unwired: 2 in, 2 out]
            }
          }
        }
        frame "Refit Curve" {
          # "Another calibration point is not required. Also  checks if there are any points to fit curve to."
        }
      }
      "Status Out" <- w480
    }
    frame #12 {
      n260 = Build Array(w683, w686, w685, w680, w684) -> (w682:dbl[][])
      n261 = call "Sort_Array_Indicies.vi"("unsorted array"=w683) -> ("Sort Index"=w679:i32[])  [unwired: 1 out]
      n262 = for {
        tunnel: w679 -> [w689]
        tunnel: w682 -> [w688] mode=indexing
        tunnel: [w687] -> w681 mode=indexing
        n263 = for {
          tunnel: w689 -> [w692] mode=indexing
          tunnel: w688 -> [w691]
          tunnel: [w690] -> w687 mode=indexing
          n264 = Index Array(array=w691, index=w692) -> (element=w690:dbl)
        }
      }
      "Ref velocity" <- w680
    }
    frame #13 {
      w700 = FALSE  # t/f
      w701 = FALSE  # t/f
      n265 = Index Array(array="Point selector 4", index=0) -> (element=w698:cluster{"Y":dbl, "Y2":dbl, "X":dbl, "t/f":bool})
      n266 = Index Array(array="Point selector 3", index=0) -> (element=w706:cluster{"Y":dbl, "X":dbl, "t/f":bool})
      n267 = Bundle By Name(cluster=w698, "t/f"=w700) -> (w699:cluster{"Y":dbl, "Y2":dbl, "X":dbl, "t/f":bool})
      n268 = Bundle By Name(cluster=w706, "t/f"=w701) -> (w702:cluster{"Y":dbl, "X":dbl, "t/f":bool})
      n269 = Build Array (concatenate)("Point selector 4", w699) -> (w695:T5)
      n270 = Build Array (concatenate)("Point selector 3", w702) -> (w704:cluster{"Y":dbl, "X":dbl, "t/f":bool}[])
      n271 = for {
        tunnel: w704 -> [w722]
        tunnel: w708 -> [w719] mode=indexing
        tunnel: [w721] -> w705 mode=indexing
        tunnel: w695 -> [w720]
        tunnel: [w718] -> w694 mode=indexing
        n272 = Index Array(array=w722, index=w719) -> (element=w721:cluster{"Y":dbl, "X":dbl, "t/f":bool})
        n273 = Index Array(array=w720, index=w719) -> (element=w718:cluster{"Y":dbl, "Y2":dbl, "X":dbl, "t/f":bool})
      }
      n274 = call "Calib_Analyse_fit.vi"("Calib file"=w709, "Input points"=w693, "polynomial order"="polynomial order", "Fixed n"="Fixed n", "n"="n", "Point selector 3"=w705, "Point selector 4"=w694) -> ("Calib const"=→"Calib const":string[][], "Calibration plot"=→"Calibration plot":cluster{cluster{dbl, dbl}[]}[], "Point selector 3 out"=w715:cluster{"Y":dbl, "X":dbl, "t/f":bool}[], "Coefficients"=→"Coefficients":dbl[][], "Point selector 4 out"=w714:T5)  [unwired: 4 out]
      n275 = local write "Point selector 3"(w715) -> ()
      n276 = local write "Point selector 4"(w714) -> ()
    }
    frame #14 {
      w738 = FALSE  # Lock File
      w740 = FALSE  # advisory dialog? (display:T)
      w741 = FALSE  # append to file? (new file:F)
      n277 = global read "Calib_global.vi" "Calib Raw Data Folder"() -> (w731:path)
      n278 = global read "Calib_global.vi" "Calib Raw Data Folder"() -> (w730:path)
      n279 = Strip Path(path=w736) -> (name=w735:string)  [unwired: 1 out]
      n280 = List Folder(path=w731) -> (filenames=w734:string[])  [unwired: 1 in, 5 out]
      n281 = Array Size(array=w734) -> (size(s)=w733:i32)
      n282 = Greater Than 0?(x=w733) -> (x > 0?=w732:bool)
      n283 = Path To String(path=w730) -> (string=w729:string)
      n284 = call "Characters_to_string.vi"("Characters to write"=w729, "Label for characters"="Calib Raw Data Folder") -> ("Output string"=w726:string)
      n285 = Concatenate Strings(w727, w726) -> (w725:string)
      n286 = global read "Calib_global.vi" "Header string"() -> (w739:string)
      n287 = call "Add_label_to_string.vi"("String to write"=w725, "File Label"="Raw data header") -> ("Output string"=w723:string)
      n288 = Concatenate Strings(w739, w723) -> (w737:string)
      n289 = case shown="True" w732 {
        tunnel: w737 -> [_ w745]
        tunnel: w735 -> [_ w744]
        tunnel: w731 -> [_ w742]
        frame False {
        }
        frame True {
          w746 = FALSE  # Lock File
          w747 = FALSE  # append to file? (new file:F)
          w748 = FALSE  # advisory dialog? (display:T)
          n290 = Build Path(base path=w742, name or relative path=w744) -> (appended path=w743:path)
          n291 = call "Write_Characters_To_File.vi"("file path (dialog if empty)"=w743, "advisory dialog? (display:T)"=w748, "character string"=w745, "append to file? (new file:F)"=w747, "Lock File"=w746) -> ()  [unwired: 4 out]
        }
      }
      n292 = call "Write_Characters_To_File.vi"("file path (dialog if empty)"=w736, "advisory dialog? (display:T)"=w740, "character string"=w737, "append to file? (new file:F)"=w741, "Lock File"=w738) -> ()  [unwired: 4 out]
    }
    frame #15 {
      n293 = case shown="\"Take new data point\"" w751 {
        tunnel: w750 -> [w754 _]
        tunnel: w749 -> [w753 _]
        frame "Take new data point" {
          n294 = global read "Calib_global.vi" "Calib Ch No"() -> (w752:string)
          n295 = stacked-sequence {
            tunnel: w754 -> [w758 w772]
            tunnel: w753 -> [_ w771]
            tunnel: w752 -> [w759 w765]
            frame #0 {
              n296 = Current VI's Path() -> (path=w761:path)
              n297 = call "Running_as_top_level.vi"("Vi path name"=w761) -> ("Top Level"=w760:bool)  [unwired: 1 out]
              n298 = case shown="True" w760 {
                frame False {
                }
                frame True {
                  n299 = call "Measurement.vi"("setup"=Setup."Setup Front Panel", "Post Process"=Post_Process."Take New Data", "File"=Save_Data."Save No Data") -> ()  [unwired: 4 in, 13 out]
                }
              }
              n300 = Build Array(w758) -> (w757:path[])
              n301 = Build Array(w759) -> (w756:string[])
              n302 = call "Current_Calib_Filenames.vi"("Calib Filename"=w757, "Channel Numbers"=w756, "Mode"=App_Global."Write to Global") -> ()  [unwired: 1 in, 2 out]
            }
            frame #1 {
              n303 = global read "Calib_global.vi" "Instrument type"() -> (w774:T13)
              n304 = case shown="\"Cross wire angle\"" w774 {
                tunnel: w765 -> [_ w782 w788]
                tunnel: [path "" ("appended path") w779 w784] -> w773
                tunnel: [FALSE TRUE TRUE] -> w768
                frame "Propeller anemometer", Default {
                }
                frame "Cross wire angle" {
                  n305 = Format Into String(format string="Ch%s_XW_Angle_Calib", w782) -> (resulting string=w778:string)  [unwired: 2 in, 1 out]
                  n306 = call "Setup_Filepath.vi"("Setup File Type"=Setup_Filetype."Calibration Setups", "Filename in"=w778) -> ("Filename Out"=w779:path)  [unwired: 1 out]
                }
                frame "Cross wire velocity" {
                  n307 = Format Into String(format string="Ch%s_XW_Velocity_Calib", w788) -> (resulting string=w785:string)  [unwired: 2 in, 1 out]
                  n308 = call "Setup_Filepath.vi"("Setup File Type"=Setup_Filetype."Calibration Setups", "Filename in"=w785) -> ("Filename Out"=w784:path)  [unwired: 1 out]
                }
              }
              n309 = Array Size(array=w771) -> (size(s)=w770:i32)
              n310 = Greater?(x=w770, y=1) -> (0:w767:bool)
              n311 = And(x=w767, y=w768) -> (x .and. y?=w766:bool)
              n312 = case shown="True" w766 {
                tunnel: w773 -> [_ w791]
                tunnel: w772 -> [_ w790]
                frame False {
                }
                frame True {
                  n313 = call "Copy_with_Check.vi"("Mode"=enum16{"Move", "Copy"}."Copy", "Target Path"=w791, "Variable Target?"=FALSE, "Source Path"=w790) -> ()  [unwired: 1 out]
                }
              }
            }
          }
        }
        frame "Refit Curve" {
        }
      }
    }
    frame #16 {
      n314 = case shown="\"Show Setup\"" w793 {
        frame "Show Setup" {
          n315 = local write "Mode"(Calib_mode."Take a New Calibration Point" ("Mode")) -> ()
        }
        frame "Take a New Calibration Point" {
        }
        frame "Refit Curve" {
        }
        frame "Setup Front Panel" {
          n316 = local write "Mode"(Calib_mode."Show Setup" ("Mode")) -> ()
        }
      }
      n317 = global write "Calib_global.vi" "Calibration Points"(dbl[] [] ("Calibration Points")) -> ()
    }
  }
